vi "Test Broken Method Error Dummy.vi"(8 "error in (no error)":errorcluster, 11 "Setup Error Test Dummy in":refnum<class "Broken Method Error Test Dummy.lvclass">) -> (0 "error out":errorcluster, 3 "Setup Error Test Dummy out":refnum<class "Broken Method Error Test Dummy.lvclass">)   [LabVIEW 2020, in "Broken Method Error Test Dummy.lvclass"]
uses:
  Broken Method Error Test Dummy.lvclass
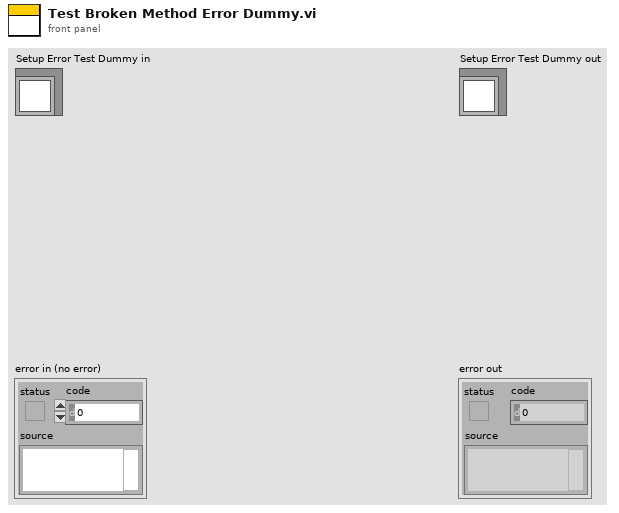
[diagram p1: front panel]
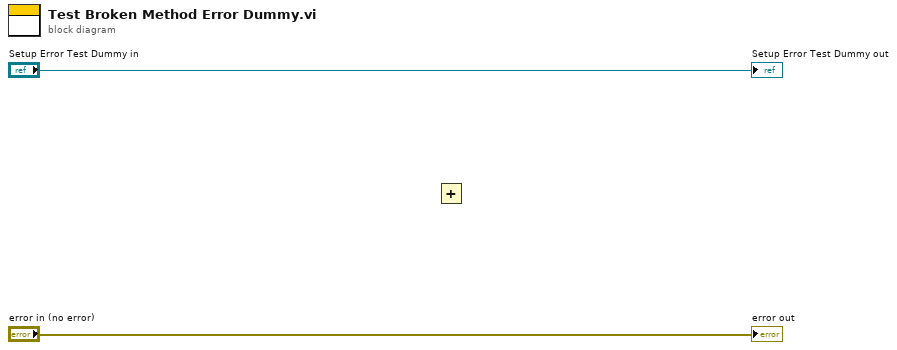
[diagram p0: block diagram]
diagram:
  n1 = Add() -> ()  [unwired: 2 in, 1 out]
  "error out" <- "error in (no error)"
  "Setup Error Test Dummy out" <- "Setup Error Test Dummy in"
